vi "Initialize Steering Frame.vi"(8 "error in (no error)":errorcluster) -> (0 "error out":errorcluster, 3 "Steering Frame out":T3)   [LabVIEW 2012]
doc: "This VI is used to initialize the mecanum and differential steering frames used to model the ROV thruster setup. The mecanum drivetrain represents the fourth thrusters that are angle tangent to the ROV's center of horizontal rotation. This allows the ROV to laterally 'crab' forward, backward, left, right and any directional vector in between. The differential drivetrain represents the two vertically pointed thrusters placed on the front and back of the ROV. This allows ROV to control its own elevation and pitch within the water.\nRuffin"
uses:
  <vilib>/robotics/Steering/Class Type Definitions/Mecanum Steering Frame.ctl
  <vilib>/robotics/Steering/Mecanum Steering Frame/NI_Robotics_Mecanum Steering Frame.lvclass
  <vilib>/robotics/Steering/Class Type Definitions/Differential Steering Frame.ctl
  <vilib>/robotics/Steering/Differential Steering Frame/NI_Robotics_Differential Steering Frame.lvclass
  <vilib>/robotics/Steering/Wheel/Wheel Parameters.ctl
  <vilib>/robotics/Steering/Wheel/Rotation Direction.ctl
  <vilib>/robotics/Steering/Mecanum Wheel/Roller Orientation.ctl
  <vilib>/robotics/Steering/Fixed Wheel/Create Fixed Wheel.vi
  <vilib>/robotics/Steering/Differential Steering Frame/Create Differential Steering Frame.vi
  <vilib>/robotics/Steering/Mecanum Wheel/Create Mecanum Wheel.vi
  <vilib>/robotics/Steering/Mecanum Steering Frame/Create Mecanum Steering Frame.vi
  <vilib>/robotics/Steering/Create Steering Frame/NI_Robotics_Create Steering Frame.xnode
  <vilib>/robotics/Steering/Class Type Definitions/NI_Robotics_Steering Class Types.lvlib
  <vilib>/robotics/Steering/Mecanum Wheel/NI_Robotics_Mecanum Wheel.lvclass
  <vilib>/robotics/Steering/Wheel/NI_Robotics_Wheel.lvclass
  <vilib>/robotics/Steering/Fixed Wheel/NI_Robotics_Fixed Wheel.lvclass
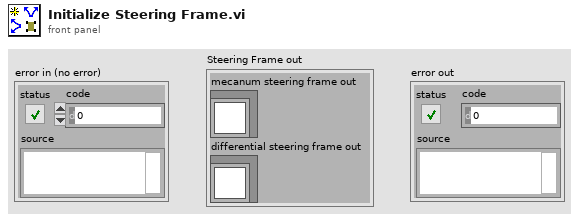
[diagram p1: front panel]
types:
  T1 = typedef "NI_Robotics_Steering Class Types.lvlib/Mecanum Steering Frame.ctl" = refnum<class "NI_Robotics_Mecanum Steering Frame.lvclass">
  T2 = typedef "NI_Robotics_Steering Class Types.lvlib/Differential Steering Frame.ctl" = refnum<class "NI_Robotics_Differential Steering Frame.lvclass">
  T3 = cluster{"mecanum steering frame out":T1, "differential steering frame out":T2}
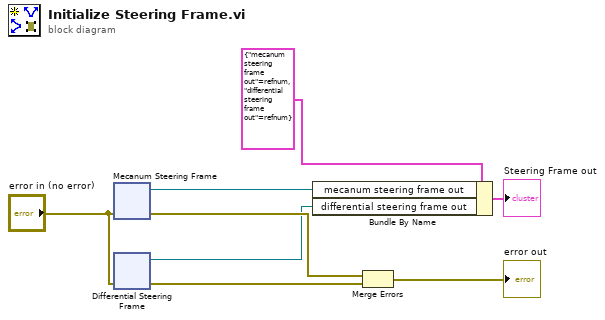
[diagram p0: block diagram]
diagram:
  n1 = xnode "Mecanum Steering Frame"("error in (no error)"="error in (no error)") -> ("mecanum steering frame out"=w3:T1, "error out"=w7:errorcluster)
  n2 = xnode "Differential Steering Frame"("error in (no error)"="error in (no error)") -> ("differential steering frame out"=w2:T2, "error out"=w6:errorcluster)
  n3 = Bundle By Name(cluster=T3 {"mecanum steering frame out"=refnum, "differential steering frame out"=refnum} ("Cluster"), "mecanum steering frame out"=w3, "differential steering frame out"=w2) -> (→"Steering Frame out":T3)
  n4 = Merge Errors(w7, w6) -> (→"error out":errorcluster)
